vi "SubVI_ReadTxt.vi"(8 "error in":errorcluster, 10 "Range Slide":cluster{dbl, dbl}={0.0, 1.0}, 11 "file path (use dialog)":path=path "D:/Desktop/A  2013-0104-1030-14.txt") -> (0 "error out":errorcluster, 1 "数组":waveform(dbl)[](array[waveform]), 2 "data":dbl[][](array[numeric]), 3 "path":path, 4 "ChannelName":string[](array[string]), 5 "dt":dbl, 6 "tend":timestamp, 7 "t0":timestamp)   [LabVIEW 2012]
uses:
  <vilib>/Waveform/WDTOps.llb/WDT Append Waveforms DBL.vi
panel:
  out "数据":waveform(dbl)
  out "数组 2":waveform(dbl)[](array[waveform])
  out "波形":waveform(dbl)
  out "x+y":timestamp
  out "波形图":waveform(dbl)[](graph)
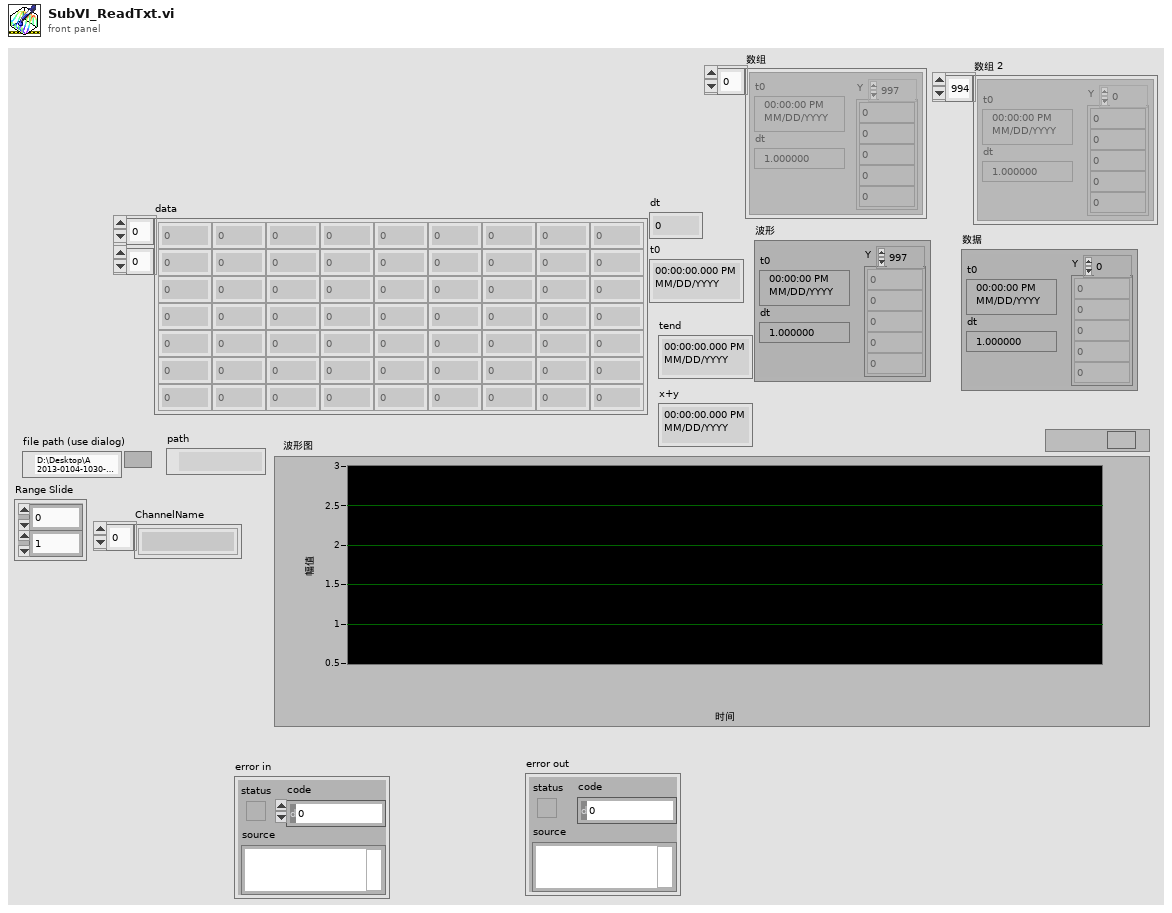
[diagram p1: front panel]
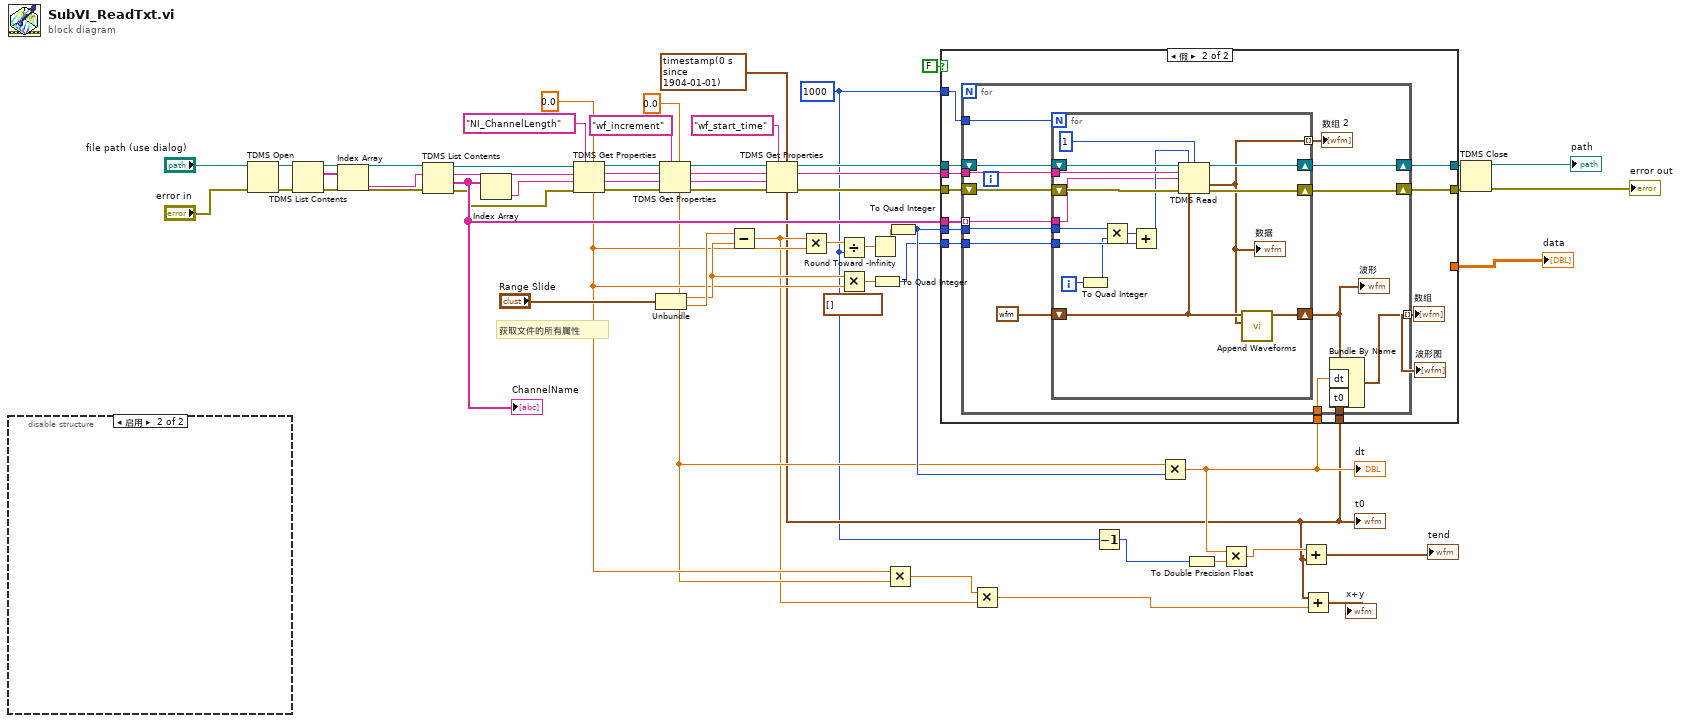
[diagram p0: block diagram]
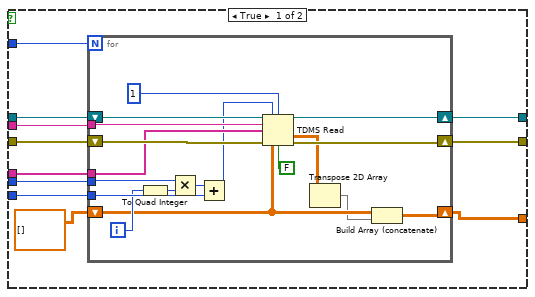
[diagram p2: hidden frame]
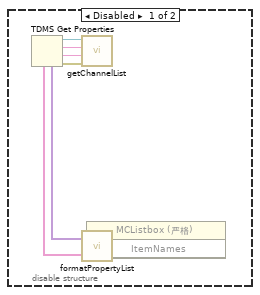
[diagram p3: hidden frame]
diagram:
  (unwired) waveform(dbl)[] []
  w4 = 1000
  # "获取文件的所有属性"
  n1 = disable-structure shown="启用" {
    frame Disabled {
      n2 = TDMS Get Properties() -> (0:w61:errorcluster, 1:w60:string, 2:w59:string, 3:w62:refnum<k34>, 4:w64:variant[], 6:w65:string[])  [unwired: 4 in, 2 out]
      n3 = call <vilib>:"getChannelList.vi"("error in (no error)"=w61, "channel names"=w60, "group name"=w59, "tdms file"=w62) -> ()  [unwired: 4 out]
      n4 = call <vilib>:"formatPropertyList.vi"("property names"=w65, "property values"=w64) -> ("strings"=w63:string[][])
      n5 = property on="属性节点" class="MCListbox (严格)"("ItemNames"=w63) -> ()  [unwired: 2 in, 2 out]
    }
    frame Enabled {
    }
  }
  n6 = TDMS Open(8:"error in", 11:"file path (use dialog)") -> (0:w37:errorcluster, 3:w38:refnum<k34>)  [unwired: 4 in]
  n7 = TDMS List Contents(4:w37, 7:w38) -> (0:w51:errorcluster, 2:w50:string[], 3:w52:refnum<k34>)  [unwired: 1 in, 1 out]
  n8 = Index Array(array=w50) -> (element=w49:string)  [unwired: 1 in]
  n9 = TDMS List Contents(4:w51, 6:w49, 7:w52) -> (0:w33:errorcluster, 1:w35:string[], 2:w36:string, 3:w34:refnum<k34>)
  "ChannelName" <- w35
  n10 = Index Array(array=w35) -> (element=w48:string)  [unwired: 1 in]
  n11 = TDMS Get Properties(5:0.0, 7:"NI_ChannelLength", 8:w33, 9:w48, 10:w36, 11:w34) -> (0:w25:errorcluster, 1:w26:string, 2:w27:string, 3:w28:refnum<k34>, 4:w13:dbl)  [unwired: 1 out]
  n12 = Unbundle("Range Slide") -> (w31:dbl, w45:dbl)
  n13 = TDMS Get Properties(5:0.0, 7:"wf_increment", 8:w25, 9:w26, 10:w27, 11:w28) -> (0:w21:errorcluster, 1:w16:string, 2:w19:string, 3:w23:refnum<k34>, 4:w12:dbl)  [unwired: 1 out]
  n14 = Subtract(x=w45, y=w31) -> (x-y=w10:dbl)
  n15 = TDMS Get Properties(5:timestamp(0 s since 1904-01-01), 7:"wf_start_time" ("属性名称"), 8:w21, 9:w16, 10:w19, 11:w23) -> (0:w20:errorcluster, 2:w18:string, 3:w22:refnum<k34>, 4:w7:timestamp)  [unwired: 2 out]
  "t0" <- w7
  n16 = Multiply(x=w10, y=w13) -> (x*y=w46:dbl)
  n17 = Divide(x=w46, y=w4) -> (x/y=w32:dbl)
  n18 = Multiply(x=w31, y=w13) -> (x*y=w44:dbl)
  n19 = Round Toward -Infinity(1:w32) -> (0:w1:dbl)
  n20 = To Quad Integer(1:w44) -> (0:w43:i64)
  n21 = Multiply(x=w13, y=w12) -> (x*y=w11:dbl)
  n22 = To Quad Integer(1:w1) -> (0:w58:i64)
  n23 = Multiply(x=w11, y=w10) -> (x*y=w6:dbl)
  n24 = Decrement(x=w4) -> (x-1=w3:i32)
  n25 = Multiply(x=w12, y=w58) -> (x*y=w9:dbl)
  "dt" <- w9
  n26 = case shown="假" FALSE {
    tunnel: w43 -> [w76 w106]
    tunnel: [w75 w105] -> w42
    tunnel: [w74 w104] -> w41
    tunnel: w35 -> [w73 w103]
    tunnel: w58 -> [w72 w102]
    tunnel: w22 -> [w71 w101]
    tunnel: w20 -> [w70 w100]
    tunnel: w18 -> [w69 w99]
    tunnel: w4 -> [w68 w98]
    tunnel: [w67 _] -> w14
    tunnel: w9 -> [_ w97]
    tunnel: w7 -> [_ w96]
    frame True {
      n27 = for {
        N: w68 -> [_]
        shift-right: [w89] -> w74
        shift-left: w71 -> [w94]
        shift-right: [w90] -> w75
        shift-left: w70 -> [w93]
        tunnel: w76 -> [w87]
        tunnel: w73 -> [w91]
        tunnel: w69 -> [w92]
        tunnel: w72 -> [w84]
        shift-right: [w82] -> w67
        shift-left: dbl[][] [] -> [w80]
        i -> [w85]
        n28 = To Quad Integer(1:w85) -> (0:w78:i64)
        n29 = Multiply(x=w84, y=w78) -> (x*y=w83:i64)
        n30 = Add(x=w83, y=w87) -> (x+y=w86:i64)
        n31 = TDMS Read(0:w94, 1:w86, 2:1, 5:w92, 7:w91, 11:w93, 12:w80, 13:FALSE ("按文件顺序返回通道？(F)")) -> (4:w89:refnum<k34>, 10:w81:dbl[][], 15:w90:errorcluster)  [unwired: 3 out]
        n32 = Transpose 2D Array(2D array=w81) -> (transposed array=w79:dbl[][])
        n33 = Build Array (concatenate)(w80, w79) -> (w82:dbl[][])
      }
    }
    frame False {
      n34 = for {
        shift-right: [w116] -> w104
        shift-left: w101 -> [w121]
        shift-right: [w117] -> w105
        shift-left: w100 -> [w120]
        tunnel: w106 -> [w115]
        tunnel: w103 -> [w118] mode=indexing
        tunnel: w99 -> [w119]
        tunnel: w102 -> [w114]
        tunnel: w98 -> [w113]
        tunnel: [w111] -> w95 mode=indexing
        tunnel: w97 -> [w110]
        tunnel: w96 -> [w109]
        n35 = for {
          N: w113 -> [_]
          tunnel: w119 -> [w135]
          tunnel: w118 -> [w126]
          tunnel: w115 -> [w131]
          tunnel: w114 -> [w129]
          shift-right: [w133] -> w116
          shift-left: w121 -> [w137]
          shift-right: [w134] -> w117
          shift-left: w120 -> [w136]
          shift-right: [w124] -> w107
          shift-left: waveform(dbl) {"t0"=timestamp(0 s since 1904-01-01), "dt"=1.0, "Y"=[]} ("波形") -> [w125]
          tunnel: [w122] -> w108 mode=indexing
          i -> [w123]
          n36 = To Quad Integer(1:w123) -> (0:w127:i64)
          n37 = Multiply(x=w129, y=w127) -> (x*y=w128:i64)
          n38 = Add(x=w128, y=w131) -> (x+y=w130:i64)
          n39 = TDMS Read(0:w137, 1:w130, 2:1, 5:w135, 7:w126, 11:w136, 12:w125) -> (4:w133:refnum<k34>, 10:w122:waveform(dbl), 15:w134:errorcluster)  [unwired: 1 in, 3 out]
          "数据" <- w122
          n40 = call-poly <vilib>:"Append Waveforms.vi"("waveform B"=w122, "waveform A"=w125) -> ("waveform out"=w124:waveform(dbl))  [unwired: 8 in, 1 out]
        }
        "波形" <- w107
        "数组 2" <- w108
        n41 = Bundle By Name(cluster=w107, "dt"=w110, "t0"=w109) -> (w111:waveform(dbl))
      }
      "数组" <- w95
      "波形图" <- w95
    }
  }
  "data" <- w14
  n42 = To Double Precision Float(number=w3) -> (double precision float=w2:dbl)
  n43 = Multiply(x=w9, y=w2) -> (x*y=w8:dbl)
  n44 = Add(x=w8, y=w7) -> (x+y=→"tend":timestamp)
  n45 = Add(x=w7, y=w6) -> (x+y=→"x+y":timestamp)
  n46 = TDMS Close(8:w42, 11:w41) -> (0:→"error out":errorcluster, 3:→"path":path)
